vi "UDP Launcher.vi"() -> ()   [LabVIEW 2022 SP3]
uses:
  UDP Input.ctl
  UDP Reader/UDP Reader/UDP Reader.lvclass
  C:/Program Files (x86)/National Instruments/LabVIEW 2022/vi.lib/ActorFramework/Actor/Actor.lvclass
  <vilib>/ActorFramework/Message Enqueuer/Message Enqueuer.lvclass/Message Enqueuer.ctl
  UDP Reader/UDP Reader Messages/Request Msg/Request Msg.lvclass/Request Msg.ctl
  <vilib>/ActorFramework/Message Enqueuer/Enqueue.vi
  <vilib>/ActorFramework/Stop Msg/Stop Msg.lvclass
  C:/Program Files (x86)/National Instruments/LabVIEW 2022/vi.lib/ActorFramework/Message/Message.lvclass
  UDP Reader/UDP Reader Messages/Request Msg/Request Msg.lvclass
  UDP Reader/UDP Reader Messages/Halt Msg/Halt Msg.lvclass
  <vilib>/ActorFramework/Message Priority Queue/Priority Enqueue.vi
  <vilib>/ActorFramework/Actor/Actor.lvclass
panel:
  in  "Input":T1={"Local IP"="", "Port"="10020", "Server IP"="224.5.23.2"}
  in  "Halt":bool
  in  "Request":bool
  in  "Stop":bool
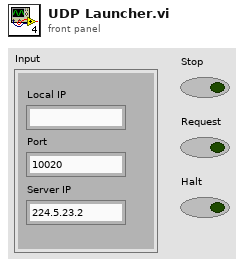
[diagram p1: front panel]
types:
  T1 = typedef "UDP Input.ctl" = cluster{"Local IP":string, "Port":string, "Server IP":string}
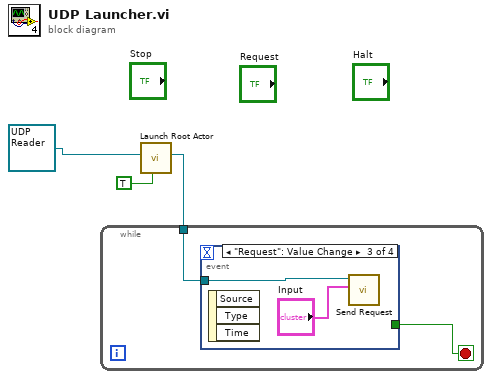
[diagram p0: block diagram]
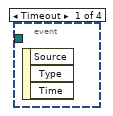
[diagram p2: hidden frame]
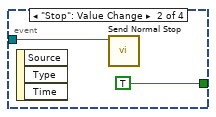
[diagram p3: hidden frame]
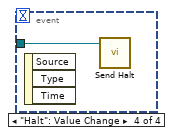
[diagram p4: hidden frame]
diagram:
  n1 = call <vilib>:"Launch Root Actor.vi"("Open Actor Core front panel? (F)"=TRUE, "Actor"=refnum<class "UDP Reader.lvclass"> refnum ("UDP Reader.lvlib:UDP Reader.lvclass")) -> ("Actor's Enqueuer"=w1:refnum<class "Message Enqueuer.lvclass">)  [unwired: 8 in, 1 out]
  n2 = while {
    tunnel: w1 -> [w5]
    stop <- w4 stop-if-true
    n3 = event shown="[2] \"Request\": Value Change" {
      selector: _ -> [_ _ _ _]
      dyn-events: _ -> [_ _ _ _]
      timeout: _ -> [_ _ _ _]
      tunnel: w5 -> [_ w7 w9 w10]
      tunnel: [_ TRUE _ _] -> w4
      event Timeout {
        n4 = event-data() -> ()  [unwired: 1 in, 3 out]
      }
      event "Stop": Value Change {
        n5 = event-data() -> ()  [unwired: 1 in, 3 out]
        n6 = call <vilib>:"Send Normal Stop.vi"("Message Enqueuer"=w7) -> ()  [unwired: 10 in, 1 out]
      }
      event "Request": Value Change {
        n7 = event-data() -> ()  [unwired: 1 in, 3 out]
        n8 = call "Send Request.vi"("Input"="Input", "Message Enqueuer in"=w9) -> ()  [unwired: 8 in, 2 out]
      }
      event "Halt": Value Change {
        n9 = event-data() -> ()  [unwired: 1 in, 3 out]
        n10 = call "Send Halt.vi"("Message Enqueuer"=w10) -> ()  [unwired: 9 in, 2 out]
      }
    }
  }
